vi "Compute Level Correction.vi"(8 "error in (no error)":errorcluster, 11 "AM in":refnum<class "AM.lvclass">) -> (0 "error out":errorcluster, 2 "Correction":dbl, 3 "AM out":refnum<class "AM.lvclass">)   [LabVIEW 2015, in "AM.lvclass"]
uses:
  AM.lvclass
  AM.lvclass/AM.ctl
  Utility VIs/Math VIs/Linear to dB (scalar).vi
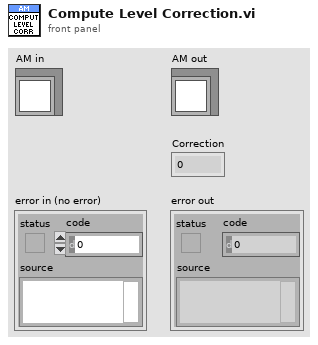
[diagram p1: front panel]
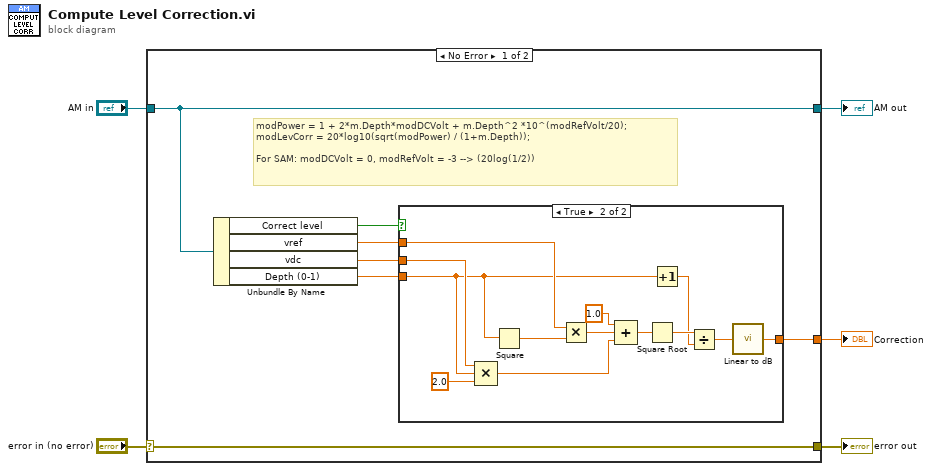
[diagram p0: block diagram]
diagram:
  n1 = case shown="No Error" "error in (no error)" {
    selector: "error in (no error)" -> [w12 w27]
    tunnel: [w12 w27] -> w4
    tunnel: [w11 w26] -> w2
    tunnel: "AM in" -> [w11 w26]
    tunnel: [w6 _] -> w1
    frame No Error {
      # "modPower = 1 + 2*m.Depth*modDCVolt + m.Depth^2 *10^(modRefVolt/20);\nmodLevCorr = 20*log10(sqrt(modPower) / (1+m.Depth));\n\nFor SAM: modDCVolt = 0, modRefVolt = -3 --> (20log(1/2))"
      n2 = Unbundle By Name(w11) -> ("Correct level"=w10:bool, "vref"=w7:dbl, "vdc"=w9:dbl, "Depth (0-1)"=w8:dbl)
      n3 = case shown="True" w10 {
        tunnel: w9 -> [_ w24]
        tunnel: w8 -> [_ w16]
        tunnel: w7 -> [_ w17]
        tunnel: [_ w13] -> w6
        frame False {
        }
        frame True {
          n4 = Compound Arithmetic op=MULTIPLY(w24, w16, 2.0 ("y")) -> (w21:dbl)
          n5 = Square(x=w16) -> (x^2=w23:dbl)
          n6 = Multiply(x=w17, y=w23) -> (x*y=w22:dbl)
          n7 = Compound Arithmetic op=ADD(1.0, w22, w21) -> (w19:dbl)
          n8 = Square Root(x=w19) -> (sqrt(x)=w18:dbl)
          n9 = Increment(x=w16) -> (x+1=w15:dbl)
          n10 = Divide(x=w18, y=w15) -> (x/y=w14:dbl)
          n11 = call-poly "Linear to dB.vi"("Linear"=w14) -> ("dB"=w13:dbl)
        }
      }
    }
    frame Error {
    }
  }
  "error out" <- w4
  "AM out" <- w2
  "Correction" <- w1
